vi "Begin.vi"(11 "Image Size":T1=enum."160x120") -> (0 "error out":errorcluster)   [LabVIEW 2011]
doc: "Called before other user functions, this VI is expected to open initial I/O refnums, load in file data, and do all program initialization. Notice that the <B>error out</B> terminal is simply used for data flow. Wiring it to other structures or subVIs ensures that this VI runs first."
uses:
  <vilib>/Rock Robotics/SystemInterfaces/DIO/FPGA_DIOPWMChannel.ctl
  <vilib>/Rock Robotics/WPI/Joystick/WPI_JoystickDeviceEnum.ctl
  <vilib>/Rock Robotics/WPI/Camera/WPI_CameraWhite Balance Values.ctl
  <vilib>/Rock Robotics/WPI/Camera/WPI_CameraExposure Values.ctl
  <vilib>/Rock Robotics/WPI/Camera/WPI_CameraFrameRate.ctl
  <vilib>/Rock Robotics/WPI/MotorControl/WPI_MotorControlOpenCANJaguar.vi
  <vilib>/Rock Robotics/WPI/CAN/Jaguar/SubVIs/WPI_CANJaguar_ControlMode.ctl
  <vilib>/Rock Robotics/WPI/RobotDrive/WPI_RobotDriveOpen2MotorWithJaguar.vi
  <vilib>/Rock Robotics/WPI/Camera/WPI_CameraImageSize.ctl
panel:
  out "error out 2":errorcluster
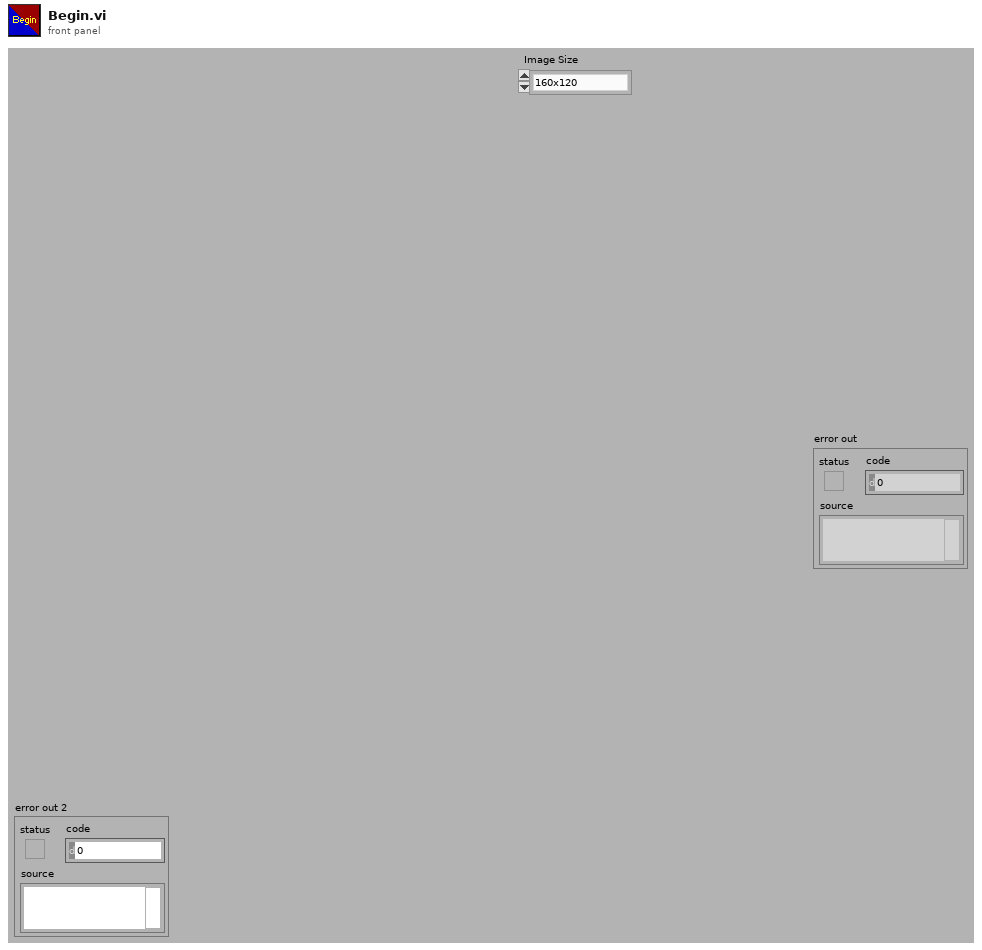
[diagram p1: front panel]
types:
  T1 = typedef "WPI_CameraImageSize.ctl" = enum16{"640x480", "320x240", "160x120"}
  T2 = typedef "WPI_CANJaguar_ControlMode.ctl" = enum8{"Percent VBus", "Current", "Speed", "Position", "Voltage"}
  T3 = typedef "WPI_JoystickDeviceEnum.ctl" = enum16{"USB 1", "USB 2", "USB 3", "USB 4", "Kinect 1", "Kinect 2"}
  T4 = typedef "WPI_CameraFrameRate.ctl" = u32
  T5 = typedef "WPI_CameraExposure Values.ctl" = enum16{"Auto", "Flicker-free 50 Hz", "Flicker-free 60 Hz", "Hold current"}
  T6 = typedef "WPI_CameraWhite Balance Values.ctl" = enum16{"Auto", "Fixed indoor", "Fixed outdoor 1", "Fixed outdoor 2", "Fixed fluorescent 1", "Fixed fluorescent 2", "Hold current"}
  T7 = typedef "FPGA_DIOPWMChannel.ctl" = enum8{"PWM 1", "PWM 2", "PWM 3", "PWM 4", "PWM 5", "PWM 6", "PWM 7", "PWM 8", "PWM 9", "PWM 10", "Invalid"}
  T8 = typedef "WPI_CameraDevRef.ctl" = cluster{"Camera Address":string, "CameraStatus":errorcluster, "Acquire Image Notifier":refnum<notifier>}
  T9 = typedef "WPI_RobotDriveDevRef.ctl" = cluster{"DevStatus":errorcluster, "Motors[]":T10[], "Square Inputs":bool, "Max Output":dbl, "Isochronous":bool}
  T10 = typedef "WPI_MotorControlDeviceRef.ctl" = cluster{"DeviceStatus":errorcluster, "Type":enum16{"PWM", "CAN"}, "PWM":cluster{"Digital Module":T11, "PWM Channel":T7, "DeadBand":T12}, "CAN":cluster{"Device Number":u8, "Control Mode":T2, "Semaphore":T13, "Max Vout":dbl}, "Invert":bool, "TransformRef":T14, "InvTransformRef":T14}
  T11 = typedef "FPGA_TypedefDigitalModule.ctl" = enum16{"Digital Module 1", "Digital Module 2"}
  T12 = typedef "WPI_PWMDeadband.ctl" = cluster{"Name":string, "maxPositivePwm":i32, "minPositivePwm":i32, "centerPwm":i32, "maxNegativePwm":i32, "minNegativePwm":i32, "angularRange":u16}
  T13 = typedef "Semaphore RefNum" = refnum<k1>
  T14 = typedef "WPI_PWMTransform_ConPane.ctl" = refnum<vi>
  T15 = typedef "WPI_JoystickDevRef.ctl" = cluster{"Device":T3}
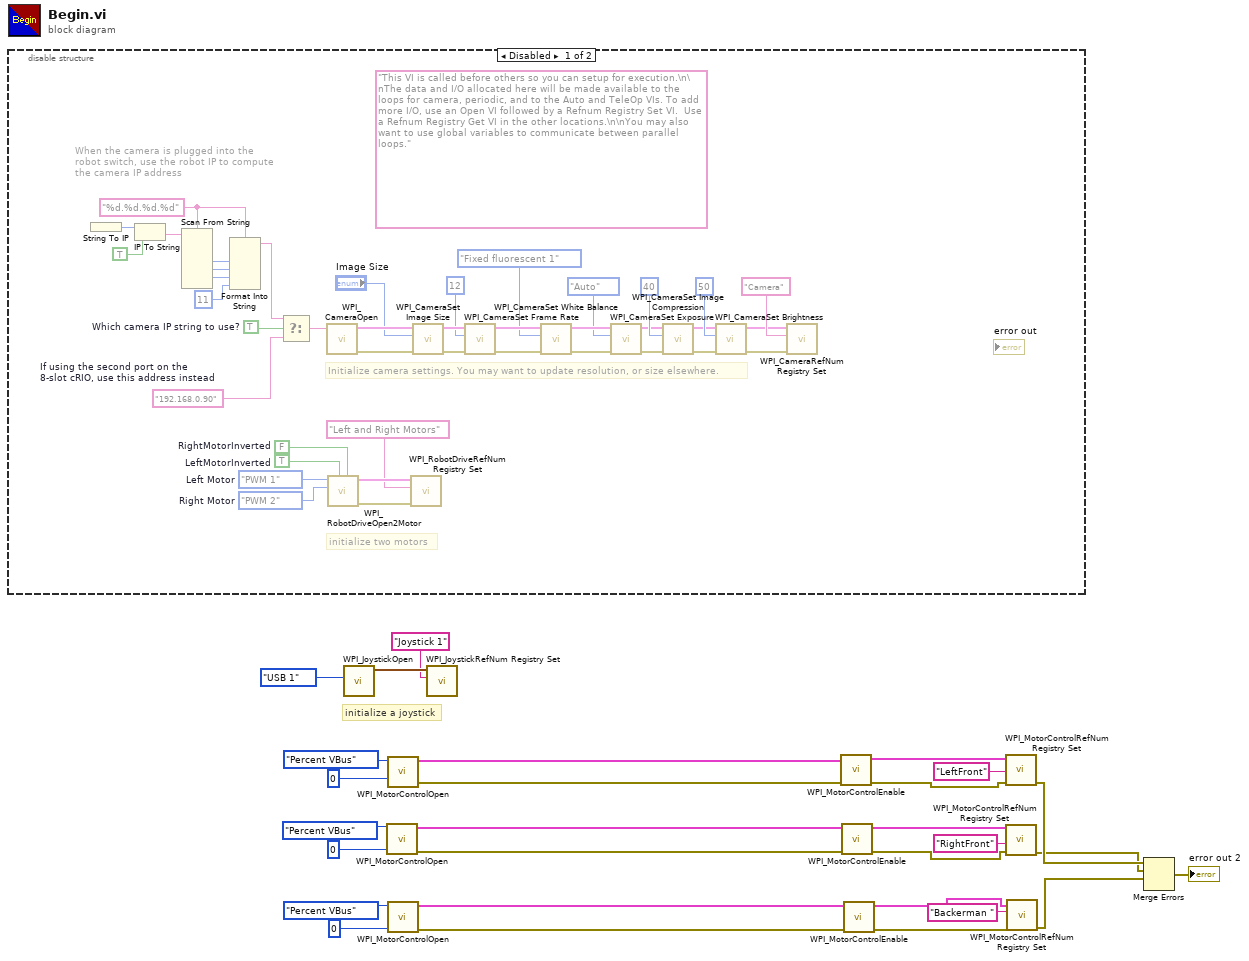
[diagram p0: block diagram]
diagram:
  # "initialize a joystick"
  n1 = disable-structure shown="Disabled" {
    frame Disabled {
      w29 = TRUE  # Which camera IP string to use?
      w33 = "%d.%d.%d.%d" ("format string")
      (unwired) "This VI is called before others so you can setup for execution.\n\nThe data and I/O allocated here will be made available to the loops for camera, periodic, and to the Auto and TeleOp VIs. To add more I/O, use an Open VI followed by a Refnum Registry Set VI.  Use a Refnum Registry Get VI in the other locations.\n\nYou may also want to use global variables to communicate between parallel loops."
      w44 = FPGA_DIOPWMChannel."PWM 2"  # Right Motor
      w45 = FPGA_DIOPWMChannel."PWM 1"  # Left Motor
      w30 = "192.168.0.90"  # If using the second port on the 8-slot cRIO, use this address instead
      w67 = TRUE  # LeftMotorInverted
      w68 = FALSE  # RightMotorInverted
      # "When the camera is plugged into the\nrobot switch, use the robot IP to compute\nthe camera IP address"
      # "initialize two motors"
      # "Initialize camera settings. You may want to update resolution, or size elsewhere."
      n2 = String To IP() -> (0:w40:u32)  [unwired: 1 in]
      n3 = IP To String(1:TRUE ("dot notation? (F)"), 2:w40) -> (0:w38:string)
      n4 = Scan From String(format string=w33, input string=w38) -> (output 1=w37:i32, output 2=w36:i32, output 3=w35:i32)  [unwired: 7 in, 3 out]
      n5 = Format Into String(format string=w33, w37, w36, w35, 11 ("Compression")) -> (resulting string=w31:string)  [unwired: 2 in, 1 out]
      n6 = Select(t=w31, s=w29, f=w30) -> (s? t:f=w32:string)
      n7 = call <vilib>:"WPI_CameraOpen.vi"("Camera Address"=w32) -> ("error out"=w54:errorcluster, "CameraDevRef"=w55:T8)  [unwired: 1 in, 8 out]
      n8 = call-poly <vilib>:"WPI_RobotDriveOpen2Motor.vi"("Right Motor Inverted"=w68, "Left Motor Inverted"=w67, "Right Motor"=w44, "Left Motor"=w45) -> ("error out"=w63:errorcluster, "RobotDriveDevRef"=w65:T9)  [unwired: 1 in, 5 out]
      n9 = call <vilib>:"WPI_RobotDriveRefNum Registry Set.vi"("error in (no error)"=w63, "refnum name"="Left and Right Motors", "RobotDriveDevRef"=w65) -> ()  [unwired: 9 out]
      n10 = call <vilib>:"WPI_CameraSet Image Size.vi"("error in (no error)"=w54, "Image Size"="Image Size", "CameraDevRef"=w55) -> ("error out"=w53:errorcluster, "CameraDevRef Out"=w56:T8)  [unwired: 7 out]
      n11 = call <vilib>:"WPI_CameraSet Frame Rate.vi"("error in (no error)"=w53, "Frame Rate (fps)"=T4 12, "CameraDevRef"=w56) -> ("error out"=w52:errorcluster, "CameraDevRef Out"=w58:T8)  [unwired: 7 out]
      n12 = call <vilib>:"WPI_CameraSet White Balance.vi"("error in (no error)"=w52, "White Balance"=WPI_CameraWhite_Balance_Values."Fixed fluorescent 1", "CameraDevRef"=w58) -> ("error out"=w51:errorcluster, "CameraDevRef Out"=w57:T8)  [unwired: 7 out]
      n13 = call <vilib>:"WPI_CameraSet Exposure.vi"("error in (no error)"=w51, "Exposure"=WPI_CameraExposure_Values."Auto", "CameraDevRef"=w57) -> ("error out"=w50:errorcluster, "CameraDevRef Out"=w60:T8)  [unwired: 7 out]
      n14 = call <vilib>:"WPI_CameraSet Image Compression.vi"("error in (no error)"=w50, "Compression"=40, "CameraDevRef"=w60) -> ("error out"=w49:errorcluster, "CameraDevRef Out"=w59:T8)  [unwired: 7 out]
      n15 = call <vilib>:"WPI_CameraSet Brightness.vi"("error in (no error)"=w49, "Brightness"=50, "CameraDevRef"=w59) -> ("error out"=w47:errorcluster, "CameraDevRef Out"=w48:T8)  [unwired: 7 out]
      n16 = call <vilib>:"WPI_CameraRefNum Registry Set.vi"("error in (no error)"=w47, "refnum name"="Camera", "CameraDevRef"=w48) -> ()  [unwired: 9 out]
    }
    frame Enabled {
    }
  }
  n17 = call <vilib>:"WPI_JoystickOpen.vi"("JoystickDevice"=WPI_JoystickDeviceEnum."USB 1") -> ("JoystickDevRef"=w28:T15)  [unwired: 10 out]
  n18 = call-poly <vilib>:"WPI_MotorControlOpen.vi"("Device Number"=u8 0, "Control Mode"=WPI_CANJaguar_ControlMode."Percent VBus") -> ("error out"=w3:errorcluster, "MotorControlDeviceRef"=w4:T10)  [unwired: 8 in]
  n19 = call-poly <vilib>:"WPI_MotorControlOpen.vi"("Device Number"=u8 0, "Control Mode"=WPI_CANJaguar_ControlMode."Percent VBus") -> ("error out"=w1:errorcluster, "MotorControlDeviceRef"=w2:T10)  [unwired: 8 in]
  n20 = call-poly <vilib>:"WPI_MotorControlOpen.vi"("Device Number"=u8 0, "Control Mode"=WPI_CANJaguar_ControlMode."Percent VBus") -> ("error out"=w12:errorcluster, "MotorControlDeviceRef"=w13:T10)  [unwired: 8 in]
  n21 = call <vilib>:"WPI_JoystickRefNum Registry Set.vi"("refnum name"="Joystick 1", "JoystickDevRef"=w28) -> ()  [unwired: 1 in, 9 out]
  n22 = call <vilib>:"WPI_MotorControlEnable.vi"("error in (no error)"=w1, "CAN Jaguar Ref"=w2) -> ("error out"=w16:errorcluster, "CAN Jaguar Ref Out"=w19:T10)  [unwired: 8 in]
  n23 = call <vilib>:"WPI_MotorControlEnable.vi"("error in (no error)"=w3, "CAN Jaguar Ref"=w4) -> ("error out"=w17:errorcluster, "CAN Jaguar Ref Out"=w18:T10)  [unwired: 8 in]
  n24 = call <vilib>:"WPI_MotorControlEnable.vi"("error in (no error)"=w12, "CAN Jaguar Ref"=w13) -> ("error out"=w15:errorcluster, "CAN Jaguar Ref Out"=w14:T10)  [unwired: 8 in]
  n25 = call <vilib>:"WPI_MotorControlRefNum Registry Set.vi"("error in (no error)"=w16, "refnum name"="LeftFront", "MotorControlDevRef"=w19) -> ("error out"=w11:errorcluster)  [unwired: 7 in, 1 out]
  n26 = call <vilib>:"WPI_MotorControlRefNum Registry Set.vi"("error in (no error)"=w17, "refnum name"="RightFront", "MotorControlDevRef"=w18) -> ("error out"=w10:errorcluster)  [unwired: 7 in, 1 out]
  n27 = call <vilib>:"WPI_MotorControlRefNum Registry Set.vi"("error in (no error)"=w15, "refnum name"="Backerman ", "MotorControlDevRef"=w14) -> ("error out"=w9:errorcluster)  [unwired: 7 in, 1 out]
  n28 = Merge Errors(w11, w10, w9) -> (→"error out 2":errorcluster)  [unwired: 1 in]
